vi "stark_decelerator.vi"() -> ()   [LabVIEW 2017, in "wf.lvlib"]
uses:
  wf.lvlib
  wf_tools/stage.ctl
  wf_channel.ctl
  <vilib>/Utility/xml.llb/Read From XML File(string).vi
  <vilib>/Utility/xml.llb/Write to XML File(string).vi
  wf_tools/wf_tools.lvlib
panel:
  in  "transmit":bool
  in  "load":bool
  in  "Save":bool
  out "init":bool
  in  "Build":bool
  in  "Stop Button":bool
  in  "Tab Control":T1(tab)
  out "electrodes":i32=109
  in  "cell length":dbl=0.005 caption="cell length (m)" format="%#_6p"
  in  "input":T2(array[cluster])=[{"final vel. (m/s)"=795.0, "distance (m)"=0.1002, "hold (s)"=1e-05}] {"hold (s)" format="%#_6p"; "distance (m)" format="%#_6p"; "final vel. (m/s)" format="%#_6p"}
  in  "initial velocity":dbl=795.0 caption="initial velocity (m/s)" format="%#_6p"
  in  "Sa / s":dbl=25000000.0 format="%#_6p"
  in  "electrodes / cell":i32=5
  out "steps":i32=3401
  out "xt":cluster{"time":dbl[], "velocity":dbl[]}[](graph)
  out "valid":bool=TRUE
  out "total d":dbl=0.10815 caption="final position (m)" format="%#_6p"
  out "total t":dbl=0.00013603773584905659 caption="total time (s)" format="%#_6p"
  out "max a":dbl caption="max accel. (m /s^2)"
  out "dt":dbl=4e-08 format="%#_6p"
  out "stages":T3[](array[typedef])=[{"v_i (m/s)"=795.0, "v_f (m/s)"=795.0, "a (m / s^2)"=0.0, "d (m)"=0.1002, "t (s)"=0.0001260377358490566}, {"v_i (m/s)"=795.0, "v_f (m/s)"=795.0, "a (m / s^2)"=0.0, "d (m)"=0.00795, "t (s)"=1e-05}] {"t (s)" format="%#_6e"; "v_i (m/s)" format="%#_6e"; "a (m / s^2)" format="%#_6e"; "d (m)" format="%#_6e"; "v_f (m/s)" format="%#_6e"}
  in  "shift":bool
  in  "delta_x":dbl=0.0001
  in  "threshold":dbl=0.1001
  in  "using":enum16{"position", "time"}(ring)
  in  "ramp tail (s)":dbl=2e-06 format="%#_6p"
  out "el":waveform(dbl)[](graph)=[{"t0"=timestamp(0 s since 1904-01-01), "dt"=4e-08, "Y"=array[3401 elements]}, {"t0"=timestamp(0 s since 1904-01-01), "dt"=4e-08, "Y"=array[3401 elements]}, {"t0"=timestamp(0 s since 1904-01-01), "dt"=4e-08, "Y"=array[3401 elements]}, {"t0"=timestamp(0 s since 1904-01-01), "dt"=4e-08, "Y"=array[3401 elements]}, {"t0"=timestamp(0 s since 1904-01-01), "dt"=4e-08, "Y"=array[3401 elements]}]
  out "el freq":waveform(dbl)(graph)={"t0"=timestamp(0 s since 1904-01-01), "dt"=4e-08, "Y"=array[3401 elements]}
  in  "ramp head (s)":dbl=4e-06 format="%#_6p"
  in  "phase_0":dbl=0.2 caption="phase_0 (/2pi)" format="%#_13g"
  in  "phase_c":dbl=-0.5 caption="phase (/ 2 pi)"
  out "corr freq":waveform(dbl)(graph)={"t0"=timestamp(0 s since 1904-01-01), "dt"=4e-08, "Y"=array[3401 elements]}
  out "corr":waveform(dbl)[](graph)=[{"t0"=timestamp(0 s since 1904-01-01), "dt"=4e-08, "Y"=array[3401 elements]}]
  in  "add func":bool=TRUE
  in  "f(x, t)":string="1000"
  in  "config":T4[](array[typedef])=[{"device"="WFG_A", "channel"=1, "Sa / s"=25000000.0, "Vpp"=5.0, "offset"=-0.0034}, {"device"="WFG_A", "channel"=2, "Sa / s"=25000000.0, "Vpp"=5.0, "offset"=-0.0013}, {"device"="WFG_B", "channel"=1, "Sa / s"=25000000.0, "Vpp"=5.0, "offset"=-0.0023}, {"device"="WFG_B", "channel"=2, "Sa / s"=25000000.0, "Vpp"=5.0, "offset"=-0.0011}, {"device"="WFG_C", "channel"=1, "Sa / s"=25000000.0, "Vpp"=5.0, "offset"=-0.0021}, {"device"="WFG_C", "channel"=2, "Sa / s"=25000000.0, "Vpp"=1.24, "offset"=0.0663}] {"Sa / s" format="%#_6p"; "channel" items=["1"=1, "2"=2]}
  # "Rydberg-Stark decelerator"
  # "Add a phase shift of [delta_x], which is triggered to occur when\n[using] > [threshold]."
  # "hardware settings for each waveform"
  # "Use the input tab to specify the electrode configuration and desired acceleration/ deceleration stages.   The electrodes are assumed to be equally spaced and grouped into cells of n electrodes, where every i'th electrode is connected to the (i + n)'th. \n\nAfter making changes to the settings ensure that the valid indicator is lit then press Build to solve the equations of motion for each stage (output to the sequence tab) and to find the position of the trap centre as a function of time.\n\nThe trap position is translated into the phase with respect to the position of each electrode, which in turn gives the electrode waveforms (these are displayed on the electrodes tab).  The waveforms can be linearly ramped on / off using the ramp head and ramp tail inputs.\n\nThe correction tab shows the waveform for the top electrode, which modulates to correct for a weakening of the trap as it passes over the regions between electrodes.  The frequency of the correction waveform is n times larger than that for the electrodes.  An arbitrary function that varies with either or both the trap position (x) and time (t) can be added to this.  This function is scaled in proportion to the amplitude of the correction function.\n\nUltimately, all of the waveforms are rescaled to be between +/- 1.\n\nTo send the waveforms to the hardware, adjust the settings on the output tab and then press Transmit. \n\nSave or Load the waveforms to a *.wf file (XML).\n\nNotes:\n - The functions of this vi are available for use as a subVI in wf_tools:create.vi\n - Loading a *.wf file will not update the input settings or frequency plots"
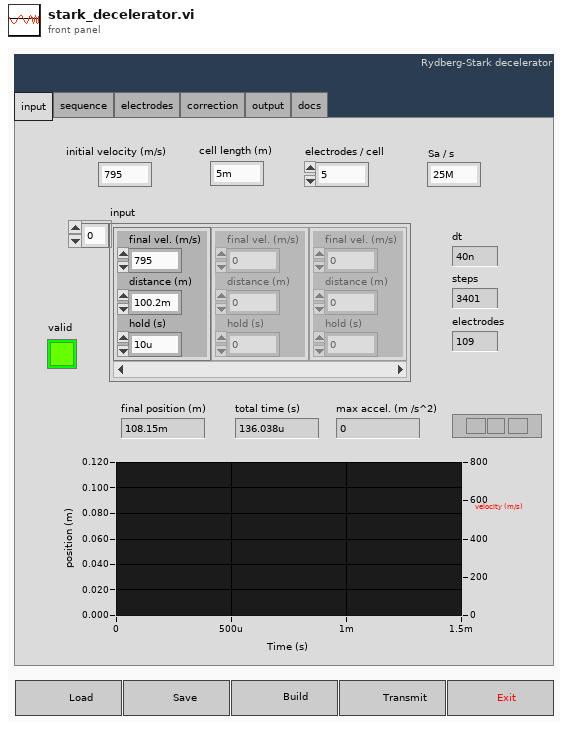
[diagram p1: front panel]
types:
  T1 = enum32{"input", "sequence", "electrodes", "correction", "output", "docs"}
  T2 = cluster{"final vel. (m/s)":dbl, "distance (m)":dbl, "hold (s)":dbl}[]
  T3 = typedef "wf.lvlib/wf_tools.lvlib/stage.ctl" = cluster{"v_i (m/s)":dbl, "v_f (m/s)":dbl, "a (m / s^2)":dbl, "d (m)":dbl, "t (s)":dbl}
  T4 = typedef "wf.lvlib/wf_channel.ctl" = cluster{"device":refnum<visa-resource-name>, "channel":u8, "Sa / s":dbl, "Vpp":dbl, "offset":dbl}
  T5 = enum8{"Enabled", "Disabled", "Disabled and Grayed Out"}
  T6 = cluster{"time":dbl[], "position":dbl[], "velocity":dbl[]}
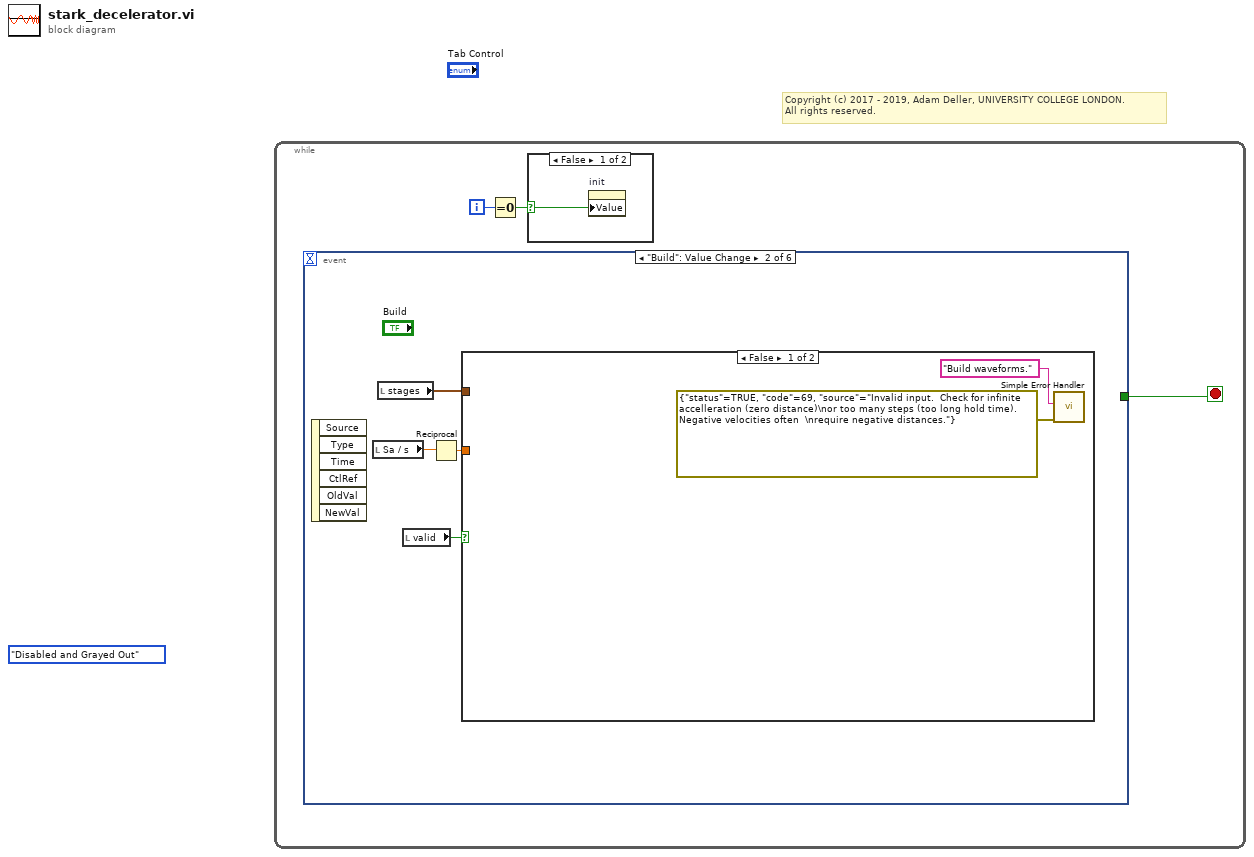
[diagram p0: block diagram]
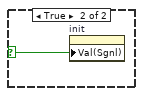
[diagram p2: hidden frame]
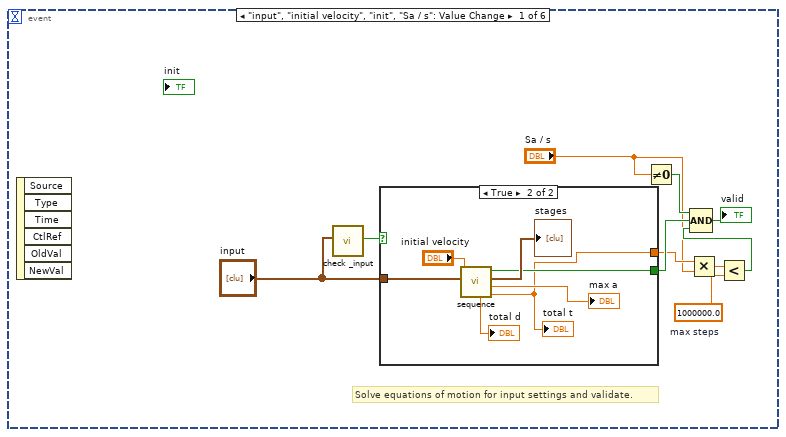
[diagram p3: hidden frame]
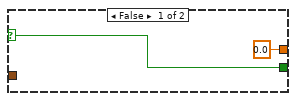
[diagram p4: hidden frame]
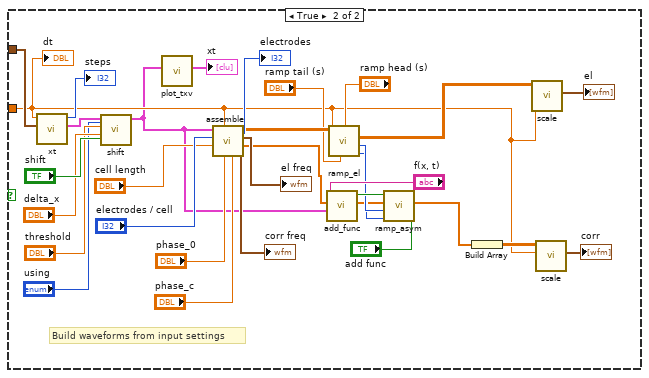
[diagram p5: hidden frame]
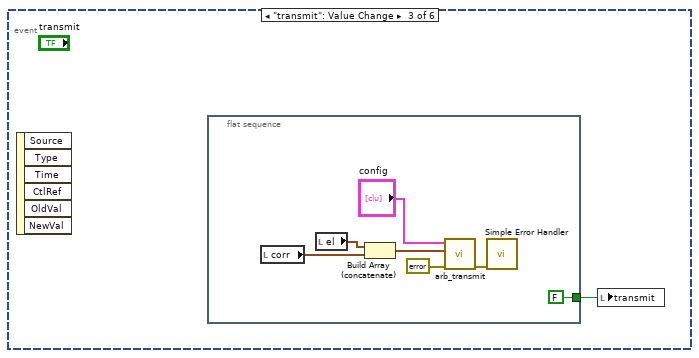
[diagram p6: hidden frame]
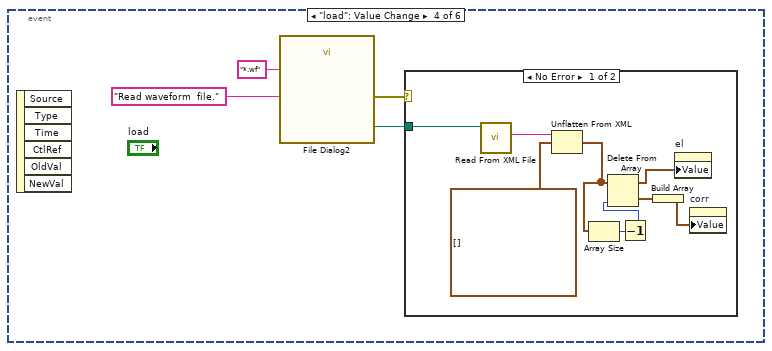
[diagram p7: hidden frame]
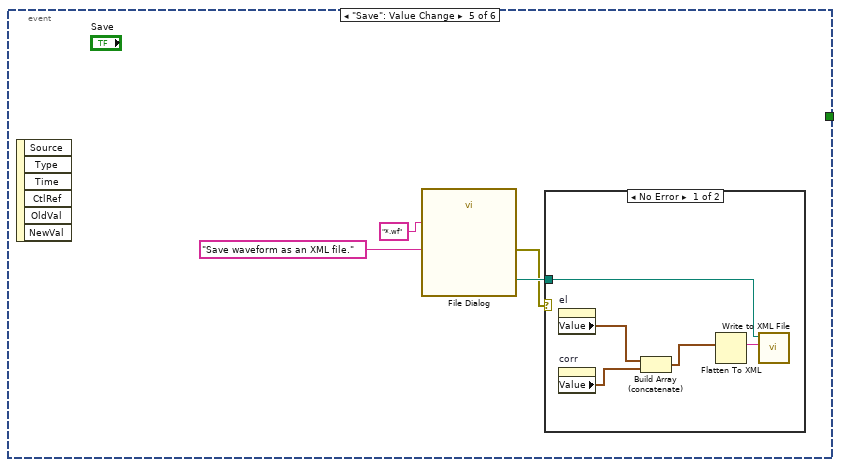
[diagram p9: hidden frame]
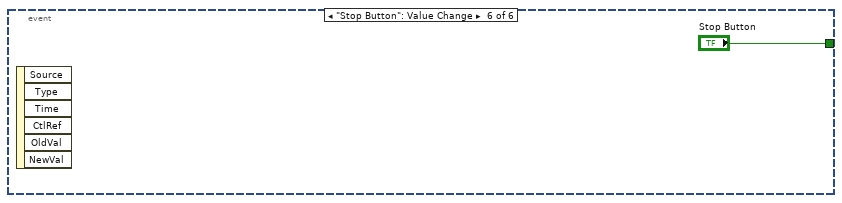
[diagram p11: hidden frame]
diagram:
  (unwired) T5."Disabled and Grayed Out" ("Disabled")
  # "Copyright (c) 2017 - 2019, Adam Deller, UNIVERSITY COLLEGE LONDON.\nAll rights reserved."
  n1 = while {
    i -> [w2]
    stop <- w3 stop-if-true
    n2 = event shown="[1] \"Build\": Value Change" {
      selector: _ -> [_ _ _ _ _ _]
      dyn-events: _ -> [_ _ _ _ _ _]
      timeout: _ -> [_ _ _ _ _ _]
      tunnel: [_ _ _ _ _ "Stop Button"] -> w3
      event "input", "initial velocity", "init", "Sa / s": Value Change {
        w8 = 1000000.0  # max steps
        # "Solve equations of motion for input settings and validate."
        n3 = event-data() -> ()  [unwired: 1 in, 6 out]
        n4 = call "check _input.vi"("input"="input") -> ("valid"=w14:bool)  [unwired: 10 in]
        n5 = case shown="True" w14 {
          selector: w14 -> [w17 _]
          tunnel: "input" -> [_ w24]
          tunnel: [w17 w21] -> w11
          tunnel: [0.0 ("total t") w18] -> w10
          frame False {
          }
          frame True {
            n6 = call "sequence.vi"("input"=w24, "initial vel."="initial velocity") -> ("total t"=w18:dbl, "max a"=→"max a":dbl, "stages"=→"stages":T3[], "valid"=w21:bool, "total d"=→"total d":dbl)  [unwired: 5 in]
            "total t" <- w18
          }
        }
        n7 = Not Equal To 0?(x="Sa / s") -> (x != 0?=w12:bool)
        n8 = Multiply(x=w10, y="Sa / s") -> (x*y=w9:dbl)
        n9 = Less?(x=w9, y=w8) -> (x < y?=w7:bool)
        n10 = Compound Arithmetic op=AND(w12, w11, w7) -> (→"valid":bool)
      }
      event "Build": Value Change {
        n11 = event-data() -> ()  [unwired: 1 in, 6 out]
        n12 = local read "Sa / s"() -> (w26:dbl)
        n13 = local read "stages"() -> (w27:T3[])
        n14 = local read "valid"() -> (w28:bool)
        n15 = Reciprocal(x=w26) -> (1/x=w25:dbl)
        n16 = case shown="False" w28 {
          tunnel: w27 -> [_ w57]
          tunnel: w25 -> [_ w41]
          frame False {
            n17 = call <vilib>:"Simple Error Handler.vi"("error source (\" \")"="Build waveforms." ("error source (\" \")"), "error in (no error)"=errorcluster {"status"=TRUE, "code"=69, "source"="Invalid input.  Check for infinite accelleration (zero distance)\nor too many steps (too long hold time). Negative velocities often  \nrequire negative distances."}) -> ()  [unwired: 3 in, 5 out]
          }
          frame True {
            # "Build waveforms from input settings"
            n18 = call "xt.vi"("stages"=w57, "dt (s)"=w41) -> ("output"=w36:T6, "num_steps"=→"steps":i32)  [unwired: 8 in]
            n19 = call "shift.vi"("shift"="shift", "using"="using", "delta_x"="delta_x", "threshold"="threshold", "txv IN"=w36) -> ("txv OUT"=w35:T6)  [unwired: 6 in]
            n20 = call "plot_txv.vi"("txv"=w35) -> ("XT"=→"xt":cluster{"time":dbl[], "velocity":dbl[]}[])  [unwired: 10 in]
            n21 = call "assemble.vi"("corr phase"="phase_c", "el phase"="phase_0", "dt"=w41, "cell length"="cell length", "electrodes/ cell"="electrodes / cell", "input"=w35) -> ("corr freq"=→"corr freq":waveform(dbl), "correction"=w40:dbl[], "el freq"=→"el freq":waveform(dbl), "electrodes"=w47:dbl[][], "num_electrodes"=→"electrodes":i32)  [unwired: 1 in]
            n22 = call "add_func.vi"("f(x, t)"="f(x, t)", "output"=w35, "wf_in"=w40, "apply"="add func") -> ("wf_out"=w38:dbl[])  [unwired: 6 in, 1 out]
            n23 = call "ramp_el.vi"("ramp tail (s)"="ramp tail (s)", "dt"=w41, "ramp head (s)"="ramp head (s)", "wf_in"=w47) -> ("num_tail"=w42:i32, "num_head"=w44:i32, "wf_out"=w46:dbl[][])  [unwired: 5 in]
            n24 = call "ramp_asym.vi"("num_tail"=w42, "num_head"=w44, "wf_in"=w38) -> ("wf_out"=w39:dbl[])  [unwired: 8 in]
            n25 = Build Array(w39) -> (w60:dbl[][])
            n26 = call "scale.vi"("dt"=w41, "waveforms"=w46) -> ("el"=→"el":waveform(dbl)[])  [unwired: 9 in]
            n27 = call "scale.vi"("dt"=w41, "waveforms"=w60) -> ("el"=→"corr":waveform(dbl)[])  [unwired: 9 in]
            "dt" <- w41
          }
        }
      }
      event "transmit": Value Change {
        n28 = event-data() -> ()  [unwired: 1 in, 6 out]
        n29 = flat-sequence {
          tunnel: [FALSE ("sending")] -> w62
          frame #0 {
            n30 = local read "corr"() -> (w67:waveform(dbl)[])
            n31 = local read "el"() -> (w66:waveform(dbl)[])
            n32 = Build Array (concatenate)(w66, w67) -> (w65:waveform(dbl)[])
            n33 = call "arb_transmit.vi"("error in (no error)"=errorcluster {"status"=FALSE, "code"=0, "source"=""}, "Waveform Graph"=w65, "output"="config") -> ("error out"=w69:errorcluster)  [unwired: 8 in]
            n34 = call <vilib>:"Simple Error Handler.vi"("error in (no error)"=w69) -> ()  [unwired: 4 in, 5 out]
          }
        }
        n35 = local write "transmit"(w62) -> ()
      }
      event "load": Value Change {
        n36 = event-data() -> ()  [unwired: 1 in, 6 out]
        n37 = call "File Dialog2"("prompt"="Read waveform  file.", "pattern (all files)"="*.wf" ("pattern label")) -> ("selected path"=w71:path, "error out"=w70:errorcluster)  [unwired: 10 in, 2 out]
        n38 = case shown="No Error" w70 {
          tunnel: w71 -> [w82 _]
          frame No Error {
            n39 = call-poly <vilib>:"Read From XML File.vi"("XML File Path"=w82) -> ("XML Elements"=w81:string)  [unwired: 8 in, 2 out]
            n40 = Unflatten From XML(xml string=w81, type=waveform(dbl)[] [] ("electrodes 2")) -> (value=w79:waveform(dbl)[])  [unwired: 1 in, 1 out]
            n41 = Array Size(array=w79) -> (size(s)=w75:i32)
            n42 = Decrement(x=w75) -> (x-1=w74:i32)
            n43 = Delete From Array(array=w79, index=w74) -> (deleted portion=w77:waveform(dbl), array with subset deleted=w78:waveform(dbl)[])  [unwired: 1 in]
            n44 = Build Array(w77) -> (w76:waveform(dbl)[])
            n45 = property on="el" class="WFGraph (strict)"("Value"=w78) -> ()  [unwired: 2 in, 2 out]
            n46 = property on="corr" class="WFGraph (strict)"("Value"=w76) -> ()  [unwired: 2 in, 2 out]
          }
          frame Error {
          }
        }
      }
      event "Save": Value Change {
        n47 = event-data() -> ()  [unwired: 1 in, 6 out]
        n48 = call "File Dialog"("prompt"="Save waveform as an XML file.", "pattern (all files)"="*.wf" ("pattern label")) -> ("selected path"=w86:path, "error out"=w83:errorcluster)  [unwired: 10 in, 2 out]
        n49 = case shown="No Error" w83 {
          tunnel: w86 -> [w90 _]
          frame No Error {
            n50 = property on="el" class="WFGraph (strict)"() -> ("Value"=w89:waveform(dbl)[])  [unwired: 2 in, 2 out]
            n51 = property on="corr" class="WFGraph (strict)"() -> ("Value"=w88:waveform(dbl)[])  [unwired: 2 in, 2 out]
            n52 = Build Array (concatenate)(w89, w88) -> (w87:waveform(dbl)[])
            n53 = Flatten To XML(anything=w87) -> (xml string=w91:string)
            n54 = call-poly <vilib>:"Write to XML File.vi"("XML Input"=w91, "XML File Path"=w90) -> ()  [unwired: 7 in, 3 out]
          }
          frame Error {
          }
        }
      }
      event "Stop Button": Value Change {
        n55 = event-data() -> ()  [unwired: 1 in, 6 out]
      }
    }
    n56 = Equal To 0?(x=w2) -> (x = 0?=w1:bool)
    n57 = case shown="False" w1 {
      selector: w1 -> [w4 w5]
      frame False {
        n58 = property on="init" class="Bool (strict)"("Value"=w4) -> ()  [unwired: 2 in, 2 out]
      }
      frame True {
        n59 = property on="init" class="Bool (strict)"("Val(Sgnl)"=w5) -> ()  [unwired: 2 in, 2 out]
      }
    }
  }
